vi "uBlaze VIVM Globals.vi"() -> ()   [LabVIEW 2011]
panel:
  out "Indicator D (+0x001C)":u32 format="%08x"
  out "Indicator C (+0x0018)":u32 format="%08x"
  out "Indicator B (+0x0014)":u32 format="%08x"
  out "Indicator A (+0x0010)":u32 format="%08x"
  in  "Control D (+0x000C)":u32 format="%08x"
  in  "Control C (+0x0008)":u32 format="%08x"
  in  "Control B (+0x0004)":u32 format="%08x"
  in  "Control A (+0x0000)":u32 format="%08x"
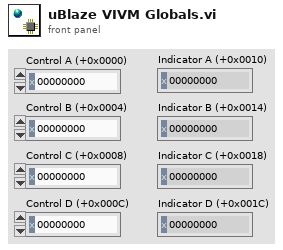
[diagram p1: front panel]
diagram:
